vi "Phasor Compute Gated Phasor.vi"(7 "Phasor Calculation Type":T1, 8 "Error In":errorcluster, 9 "j 2 pi f":cxt, 10 "Gates Definitions":T4={"First Gate: t1"=0.0, "Gate Width: W"=0.0, "Gate Step: d"=0.0, "# Gates: G"=0.0, "Use Gate Center"=FALSE, "Frames/Image: F"=50, "Gates/Frame: L"=0, "Bits/Frame: q"=0, "Multiplicity: p"=0, "Gate Type"=enum."Square", "Gate Edge s"=4.0, "Gate Top Slope"=4.0, "Reversed Sawtooth?"=FALSE, "Computation"=FALSE, "User-defined Gate"={"X Array"=[], "Y Array"=[]}, "Tolerance"=50.0, "Integration"=enum."Item 0", "# Steps"=50.0, "Type of User-defined Function"=enum."Gate"}, 11 "Decay Definition":T2={"offset: t0"=0.0, "period: T"=0.0, "lifetime: tau"=0.0, "Incident Signal: I"=0.5, "Normalized Decays"=FALSE, "IRF Model"=enum."Dirac", "IRF Parameter 1"=0.0, "Poisson Signal"=FALSE}) -> (0 "Error Out":errorcluster, 3 "phasor":cxt, 4 "CPU (s)":dbl)   [LabVIEW 2021, in "Phasor.lvlib"]
uses:
  Phasor.lvlib
  Phasor Gate Definitions.ctl
  Phasor Gate Type.ctl
  Graphs/XY Graph/XY Graph Plot Data.ctl
  Phasor Decay Definiton.ctl
  Phasor IRF Model.ctl
  Phasor Calculation Type.ctl
  013d9567-a06e-4633-918d-fb7b214fbd4f.vi
  a72c2c01-1e7c-47d2-97e3-0247e5e3b51b.vi
  5bfd5da1-96d5-4f5c-8101-185aed7e9c89.vi
  a72c2c01-1e7c-47d2-97e3-0247e5e3b51b.vi/8a80743f-1319-44c8-96b0-3ef8fc688731.vi
  a72c2c01-1e7c-47d2-97e3-0247e5e3b51b.vi/931f4f8f-d8c6-4056-833f-5c8fe97b24b9.vi
  Math/ix/ix (EXT).vi
  Math/Math.lvlib
  Graphs/XY Graph/XY Graph Add-Ons.lvlib
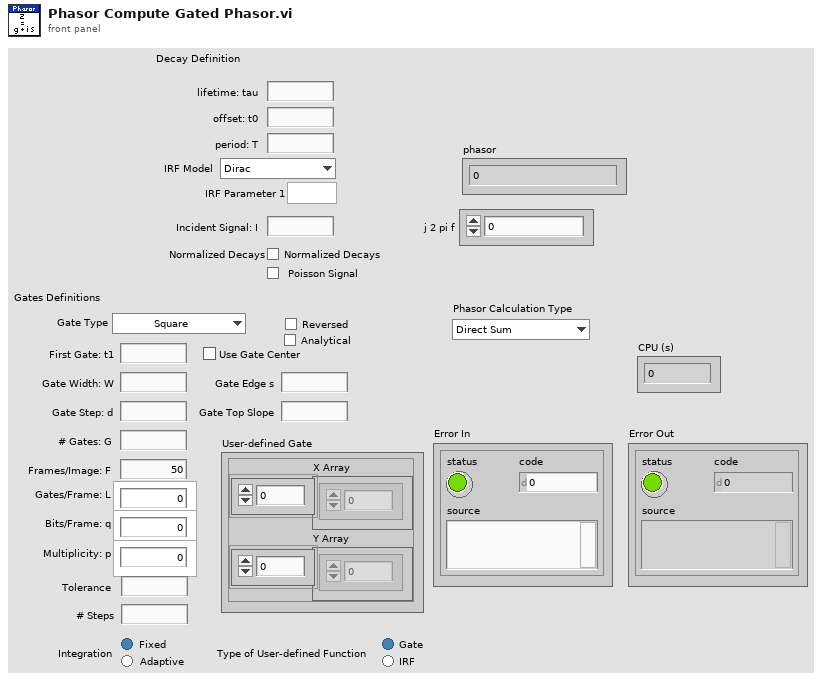
[diagram p1: front panel]
types:
  T1 = typedef "Phasor.lvlib/Phasor Calculation Type.ctl" = enum16{"Direct Sum", "Analytical Formula"}
  T2 = typedef "Phasor.lvlib/Phasor Decay Definiton.ctl" = cluster{"offset: t0":ext, "period: T":ext, "lifetime: tau":ext, "Incident Signal: I":ext, "Normalized Decays":bool, "IRF Model":T3, "IRF Parameter 1":ext, "Poisson Signal":bool}
  T3 = typedef "Phasor.lvlib/Phasor IRF Model.ctl" = enum16{"Dirac", "Exponential"}
  T4 = typedef "Phasor.lvlib/Phasor Gate Definitions.ctl" = cluster{"First Gate: t1":ext, "Gate Width: W":ext, "Gate Step: d":ext, "# Gates: G":ext, "Use Gate Center":bool, "Frames/Image: F":i32, "Gates/Frame: L":i32, "Bits/Frame: q":i32, "Multiplicity: p":i32, "Gate Type":T5, "Gate Edge s":ext, "Gate Top Slope":ext, "Reversed Sawtooth?":bool, "Computation":bool, "User-defined Gate":T6, "Tolerance":ext, "Integration":enum32{"Item 0", "Item 1"}, "# Steps":ext, "Type of User-defined Function":enum32{"Gate", "IRF"}}
  T5 = typedef "Phasor.lvlib/Phasor Gate Type.ctl" = enum16{"Square", "Finite Edge Square", "Finite Edge, Tilted Top Square", "Triangle", "Sawtooth", "User-defined"}
  T6 = typedef "XY Graph Add-Ons.lvlib/XY Graph Plot Data.ctl" = cluster{"X Array":dbl[], "Y Array":dbl[]}
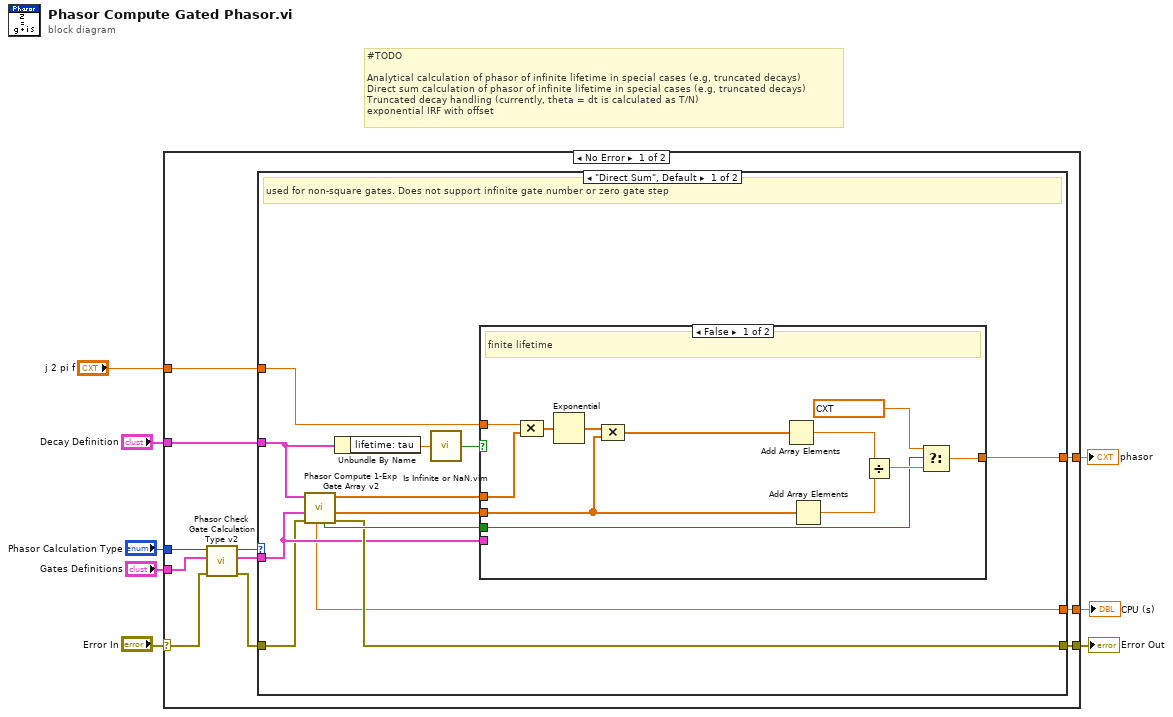
[diagram p0: block diagram]
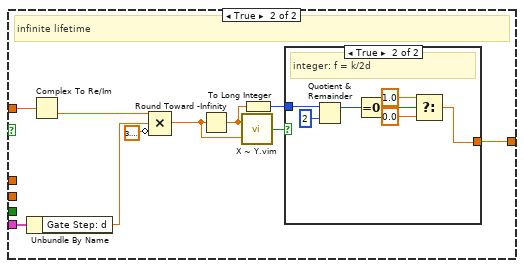
[diagram p2: hidden frame]
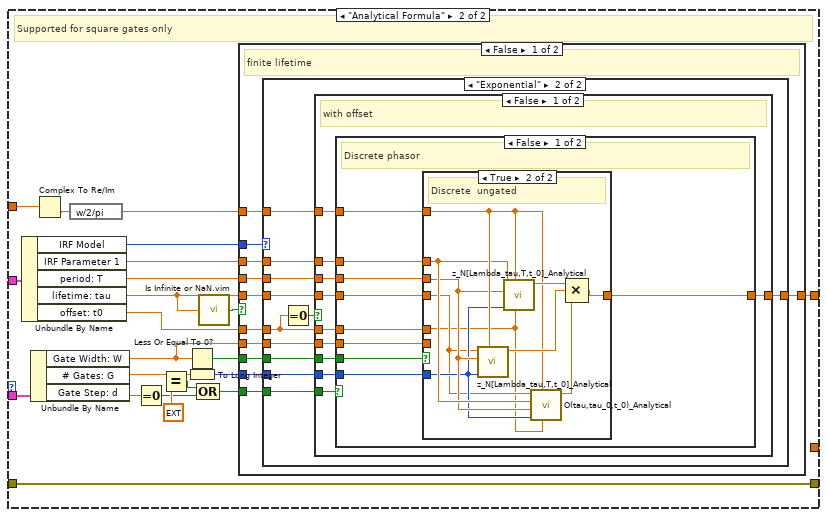
[diagram p4: hidden frame]
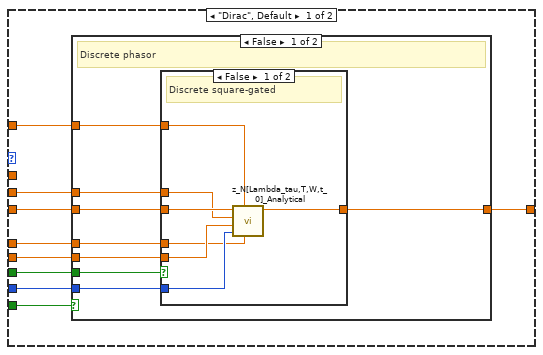
[diagram p5: hidden frame]
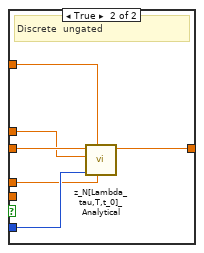
[diagram p6: hidden frame]
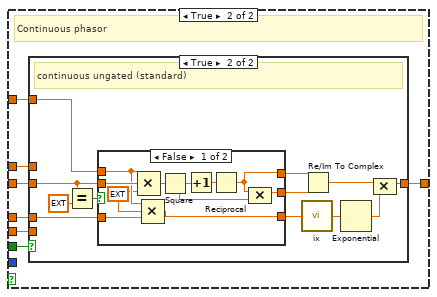
[diagram p7: hidden frame]
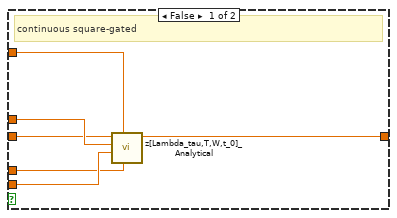
[diagram p8: hidden frame]
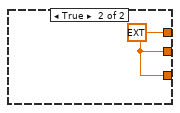
[diagram p9: hidden frame]
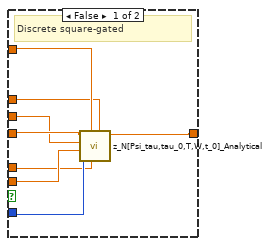
[diagram p10: hidden frame]
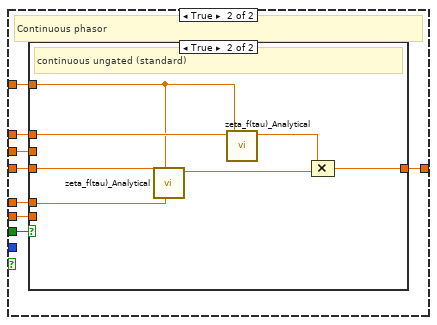
[diagram p11: hidden frame]
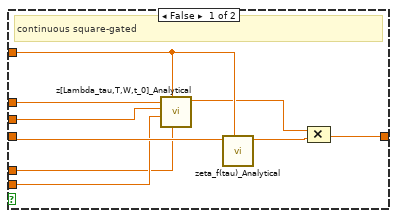
[diagram p12: hidden frame]
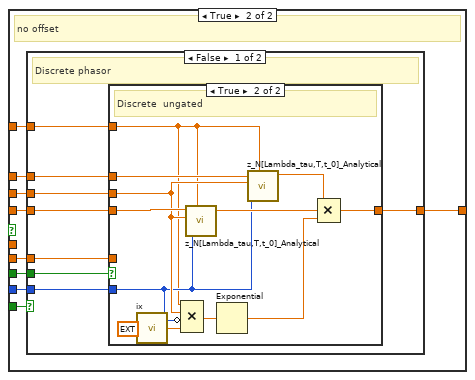
[diagram p13: hidden frame]
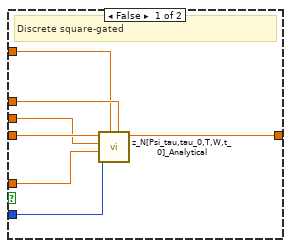
[diagram p14: hidden frame]
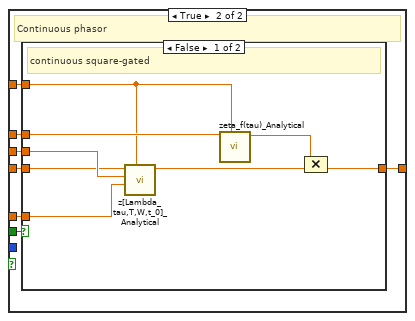
[diagram p15: hidden frame]
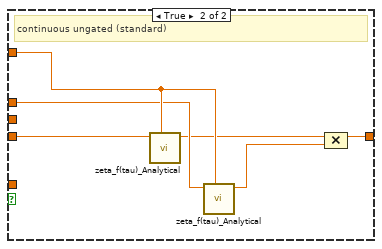
[diagram p16: hidden frame]
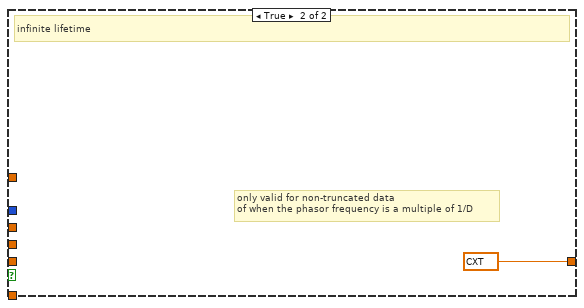
[diagram p17: hidden frame]
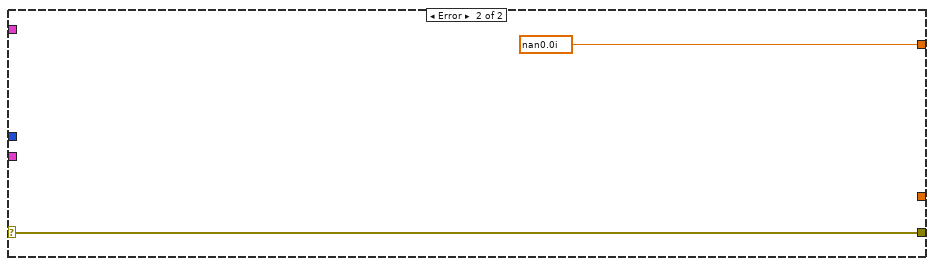
[diagram p18: hidden frame]
diagram:
  # "#TODO\n\nAnalytical calculation of phasor of infinite lifetime in special cases (e.g, truncated decays)\nDirect sum calculation of phasor of infinite lifetime in special cases (e.g, truncated decays)\nTruncated decay handling (currently, theta = dt is calculated as T/N)\nexponential IRF with offset"
  n1 = case shown="No Error" "Error In" {
    selector: "Error In" -> [w12 w291]
    tunnel: "Gates Definitions" -> [w13 _]
    tunnel: [w19 cdb nan+0.0i ("z")] -> w7
    tunnel: "Decay Definition" -> [w18 _]
    tunnel: "j 2 pi f" -> [w17 _]
    tunnel: "Phasor Calculation Type" -> [w14 _]
    tunnel: [w16 w291] -> w2
    tunnel: [w9 _] -> w1
    frame No Error {
      n2 = call "Phasor Check Gate Calculation Type v2.vi"("Error In"=w12, "Gates Definitions in"=w13, "Phasor Calculation Type in"=w14) -> ("Error Out"=w10:errorcluster, "Gates Definitions out"=w11:T4, "Phasor Calculation Type out"=w15:T1)  [unwired: 6 in]
      n3 = case shown="\"Direct Sum\", Default" w15 {
        tunnel: [w28 w78] -> w19
        tunnel: w18 -> [w24 w81]
        tunnel: w17 -> [w29 w80]
        tunnel: [w23 w61] -> w16
        tunnel: w11 -> [w22 w62]
        tunnel: w10 -> [w21 w61]
        tunnel: [w20 _] -> w9
        frame "Direct Sum", Default {
          # "used for non-square gates. Does not support infinite gate number or zero gate step"
          n4 = call "Phasor Compute 1-Exp Gate Array v2.vi"("Error In"=w21, "Gates Definitions"=w22, "Decay Definition"=w24) -> ("Error Out"=w23:errorcluster, "Gate Image Array"=w31:ext[], "t Array"=w30:ext[], "Small Gate Values?"=w27:bool, "CPU (s)"=w20:dbl)  [unwired: 4 in]
          n5 = Unbundle By Name(w24) -> ("lifetime: tau"=w26:ext)
          n6 = call "Is Infinite or NaN.vim"("Number"=w26) -> ("Is NaN or Inf?"=w25:bool)  [unwired: 8 in]
          n7 = case shown="False" w25 {
            tunnel: w31 -> [w41 _]
            tunnel: w30 -> [w38 _]
            tunnel: w29 -> [w37 w52]
            tunnel: [w35 w44] -> w28
            tunnel: w27 -> [w33 _]
            tunnel: w22 -> [_ w53]
            frame False {
              # "finite lifetime"
              n8 = Compound Arithmetic op=MULTIPLY(w37, w38) -> (w39:cxt[])
              n9 = Exponential(1:w39) -> (0:w40:cxt[])
              n10 = Compound Arithmetic op=MULTIPLY(w40, w41) -> (w36:cxt[])
              n11 = Add Array Elements(numeric array=w36) -> (sum=w42:cxt)
              n12 = Add Array Elements(numeric array=w41) -> (sum=w43:ext)
              n13 = Divide(x=w42, y=w43) -> (x/y=w34:cxt)
              n14 = Select(t=cxt nan+nani, s=w33, f=w34) -> (s? t:f=w35:cxt)
            }
            frame True {
              # "infinite lifetime"
              n15 = Unbundle By Name(w53) -> ("Gate Step: d"=w50:ext)
              n16 = Complex To Re/Im(x + iy=w52) -> (y=w51:ext)  [unwired: 1 out]
              n17 = Compound Arithmetic op=MULTIPLY(w51, w50, invert 3.141592653589793) -> (w48:ext)
              n18 = Round Toward -Infinity(1:w48) -> (0:w46:ext)
              n19 = call "X ~ Y.vim"("X"=w46, "Y"=w48) -> ("X ~= Y?"=w47:bool)  [unwired: 13 in]
              n20 = To Long Integer(number=w46) -> (32bit integer=w45:i32)
              n21 = case shown="True" w47 {
                tunnel: w45 -> [_ w60]
                tunnel: [_ w54] -> w44
                frame False {
                  # "not integer: f != k/2d"
                }
                frame True {
                  # "integer: f = k/2d"
                  n22 = Quotient & Remainder(x=w60, y=2) -> (x-y*floor(x/y)=w58:i32)  [unwired: 1 out]
                  n23 = Equal To 0?(x=w58) -> (x = 0?=w57:bool)
                  n24 = Select(t=1.0, s=w57, f=0.0) -> (s? t:f=w54:dbl)
                }
              }
            }
          }
        }
        frame "Analytical Formula" {
          # "Supported for square gates only"
          n25 = Unbundle By Name(w81) -> ("IRF Model"=w70:T3, "IRF Parameter 1"=w69:ext, "period: T"=w79:ext, "lifetime: tau"=w72:ext, "offset: t0"=w75:ext)
          n26 = Unbundle By Name(w62) -> ("Gate Width: W"=w77:ext, "# Gates: G"=w67:ext, "Gate Step: d"=w68:ext)
          n27 = Complex To Re/Im(x + iy=w80) -> (y=w73:ext)  [unwired: 1 out]
          n28 = expression code="w/2/pi"(w73) -> (w74:ext)
          n29 = Equal To 0?(x=w68) -> (x = 0?=w64:bool)
          n30 = Equal?(x=w67, y=ext inf) -> (x = y?=w65:bool)
          n31 = Less Or Equal To 0?(x=w77) -> (x <= 0?=w82:bool)
          n32 = To Long Integer(number=w67) -> (32bit integer=w76:i32)
          n33 = Compound Arithmetic op=OR(w65, w64) -> (w63:bool)
          n34 = call "Is Infinite or NaN.vim"("Number"=w72) -> ("Is NaN or Inf?"=w71:bool)  [unwired: 8 in]
          n35 = case shown="False" w71 {
            tunnel: w82 -> [w93 _]
            tunnel: w79 -> [w92 _]
            tunnel: [w91 cxt 0.0+0.0i ("z")] -> w78
            tunnel: w77 -> [w90 _]
            tunnel: w76 -> [w89 _]
            tunnel: w75 -> [w88 _]
            tunnel: w74 -> [w87 _]
            tunnel: w72 -> [w86 _]
            tunnel: w70 -> [w84 _]
            tunnel: w69 -> [w83 _]
            tunnel: w63 -> [w85 _]
            frame False {
              # "finite lifetime"
              n36 = case shown="\"Exponential\"" w84 {
                tunnel: w93 -> [w102 w170]
                tunnel: w92 -> [w101 w169]
                tunnel: [w100 w168] -> w91
                tunnel: w90 -> [w99 w167]
                tunnel: w89 -> [w98 w166]
                tunnel: w88 -> [w97 w161]
                tunnel: w87 -> [w96 w165]
                tunnel: w86 -> [w95 w164]
                tunnel: w85 -> [w94 w163]
                tunnel: w83 -> [_ w162]
                frame "Dirac", Default {
                  n37 = case shown="False" w94 {
                    tunnel: w102 -> [w110 w130]
                    tunnel: w96 -> [w107 w129]
                    tunnel: w101 -> [w108 w126]
                    tunnel: w95 -> [w109 w128]
                    tunnel: [w106 w127] -> w100
                    tunnel: w99 -> [w104 w125]
                    tunnel: w98 -> [w105 _]
                    tunnel: w97 -> [w103 w124]
                    frame False {
                      # "Discrete phasor"
                      n38 = case shown="False" w110 {
                        tunnel: w109 -> [w117 w123]
                        tunnel: w108 -> [w116 w122]
                        tunnel: w107 -> [w112 w119]
                        tunnel: [w113 w121] -> w106
                        tunnel: w105 -> [w114 w120]
                        tunnel: w104 -> [w115 _]
                        tunnel: w103 -> [w111 w118]
                        frame False {
                          # "Discrete square-gated"
                          n39 = call "z_N[Lambda_tau,T,W,t_0]_Analytical.vi"("t0"=w111, "Harmonic f"=w112, "N"=w114, "W"=w115, "T"=w116, "tau"=w117) -> ("z_n,N,W(tau)"=w113:cxt)  [unwired: 5 in]
                        }
                        frame True {
                          # "Discrete  ungated"
                          n40 = call "z_N[Lambda_tau,T,t_0]_Analytical.vi"("t0"=w118, "Harmonic f"=w119, "N"=w120, "T"=w122, "tau"=w123) -> ("z"=w121:cxt)  [unwired: 6 in]
                        }
                      }
                    }
                    frame True {
                      # "Continuous phasor"
                      n41 = case shown="True" w130 {
                        tunnel: w129 -> [w131 w148]
                        tunnel: w128 -> [w135 w141]
                        tunnel: [w133 w143] -> w127
                        tunnel: w126 -> [w136 _]
                        tunnel: w125 -> [w134 _]
                        tunnel: w124 -> [w132 w144]
                        frame False {
                          # "continuous square-gated"
                          n42 = call "z[Lambda_tau,T,W,t_0]_Analytical.vi"("t0"=w132, "Harmonic f"=w131, "W"=w134, "T"=w136, "tau"=w135) -> ("z"=w133:cxt)  [unwired: 6 in]
                        }
                        frame True {
                          # "continuous ungated (standard)"
                          n43 = Equal?(x=w141, y=ext inf) -> (x = y?=w138:bool)
                          n44 = case shown="False" w138 {
                            tunnel: [w151 w159] -> w147
                            tunnel: [w149 w159] -> w146
                            tunnel: w148 -> [w155 _]
                            tunnel: w141 -> [w158 _]
                            tunnel: w144 -> [w153 _]
                            tunnel: [w152 w159] -> w139
                            frame False {
                              w154 = ext 6.283185307179586477
                              n45 = Compound Arithmetic op=MULTIPLY(w155, w158, w154) -> (w150:ext)
                              n46 = Compound Arithmetic op=MULTIPLY(w155, w154, w153) -> (w152:ext)
                              n47 = Square(x=w150) -> (x^2=w157:ext)
                              n48 = Increment(x=w157) -> (x+1=w156:ext)
                              n49 = Reciprocal(x=w156) -> (1/x=w151:ext)
                              n50 = Compound Arithmetic op=MULTIPLY(w151, w150) -> (w149:ext)
                            }
                            frame True {
                              w159 = ext 0.0 ("Re")
                              # "tau = Inf"
                            }
                          }
                          n51 = call-poly "ix.vi"("x (1)"=w139) -> ("i.(x)"=w137:cxt)
                          n52 = Re/Im To Complex(1:w146, 2:w147) -> (0:w145:cxt)
                          n53 = Exponential(1:w137) -> (0:w142:cxt)
                          n54 = Compound Arithmetic op=MULTIPLY(w145, w142) -> (w143:cxt)
                        }
                      }
                    }
                  }
                }
                frame "Exponential" {
                  n55 = Equal To 0?(x=w161) -> (x = 0?=w160:bool)
                  n56 = case shown="False" w160 {
                    tunnel: w170 -> [w175 w240]
                    tunnel: w169 -> [w179 w239]
                    tunnel: [w173 w238] -> w168
                    tunnel: w167 -> [w176 w237]
                    tunnel: w166 -> [w172 w236]
                    tunnel: w165 -> [w180 w235]
                    tunnel: w164 -> [w178 w234]
                    tunnel: w163 -> [w174 w233]
                    tunnel: w162 -> [w171 w232]
                    tunnel: w161 -> [w177 _]
                    frame False {
                      # "with offset"
                      n57 = case shown="False" w174 {
                        tunnel: w175 -> [w189 w215]
                        tunnel: w180 -> [w186 w214]
                        tunnel: w179 -> [w187 w211]
                        tunnel: w178 -> [w188 w213]
                        tunnel: [w181 w212] -> w173
                        tunnel: w176 -> [w184 w210]
                        tunnel: w172 -> [w185 _]
                        tunnel: w177 -> [w183 w209]
                        tunnel: w171 -> [w182 w208]
                        frame False {
                          # "Discrete phasor"
                          n58 = case shown="True" w189 {
                            tunnel: w188 -> [w195 w199]
                            tunnel: w187 -> [w194 w201]
                            tunnel: w186 -> [w197 w203]
                            tunnel: w185 -> [w192 w200]
                            tunnel: w184 -> [w193 _]
                            tunnel: w183 -> [w191 w198]
                            tunnel: w182 -> [w196 w202]
                            tunnel: [w190 w205] -> w181
                            frame False {
                              # "Discrete square-gated"
                              n59 = call "z_N[Psi_tau,tau_0,T,W,t_0]_Analytical.vi"("tau_0"=w196, "t0"=w191, "Harmonic f"=w197, "N"=w192, "W"=w193, "T"=w194, "tau"=w195) -> ("z_n,N,W(tau,tau_0)"=w190:cxt)  [unwired: 4 in]
                            }
                            frame True {
                              # "Discrete  ungated"
                              n60 = call "z_N[Lambda_tau,T,t_0]_Analytical.vi"("Harmonic f"=w203, "N"=w200, "T"=w201, "tau"=w199) -> ("z"=w206:cxt)  [unwired: 7 in]
                              n61 = call "z_N[Lambda_tau,T,t_0]_Analytical.vi"("t0"=w198, "Harmonic f"=w203, "N"=w200, "T"=w201, "tau"=w202) -> ("z"=w207:cxt)  [unwired: 6 in]
                              n62 = call "O(tau,tau_0,t_0)_Analytical.vi"("t0"=w198, "Harmonic f"=w203, "N"=w200, "T"=w201, "tau_0"=w202, "tau"=w199) -> ("O(tau_tau_0,t_0)"=w204:cxt)  [unwired: 5 in]
                              n63 = Compound Arithmetic op=MULTIPLY(w207, w206, w204) -> (w205:cxt)
                            }
                          }
                        }
                        frame True {
                          # "Continuous phasor"
                          n64 = case shown="True" w215 {
                            tunnel: w214 -> [w222 w228]
                            tunnel: w213 -> [w224 w227]
                            tunnel: [w216 w230] -> w212
                            tunnel: w211 -> [w220 _]
                            tunnel: w210 -> [w219 _]
                            tunnel: w209 -> [w218 w225]
                            tunnel: w208 -> [w221 w229]
                            frame False {
                              # "continuous square-gated"
                              n65 = call "z[Lambda_tau,T,W,t_0]_Analytical.vi"("t0"=w218, "Harmonic f"=w222, "W"=w219, "T"=w220, "tau"=w221) -> ("z"=w217:cxt)  [unwired: 6 in]
                              n66 = call "zeta_f(tau)_Analytical.vi"("Harmonic f"=w222, "tau"=w224) -> ("z"=w223:cxt)  [unwired: 9 in]
                              n67 = Compound Arithmetic op=MULTIPLY(w217, w223) -> (w216:cxt)
                            }
                            frame True {
                              # "continuous ungated (standard)"
                              n68 = call "zeta_f(tau)_Analytical.vi"("t0"=w225, "Harmonic f"=w228, "tau"=w227) -> ("z"=w226:cxt)  [unwired: 8 in]
                              n69 = call "zeta_f(tau)_Analytical.vi"("Harmonic f"=w228, "tau"=w229) -> ("z"=w231:cxt)  [unwired: 9 in]
                              n70 = Compound Arithmetic op=MULTIPLY(w231, w226) -> (w230:cxt)
                            }
                          }
                        }
                      }
                    }
                    frame True {
                      # "no offset"
                      n71 = case shown="False" w233 {
                        tunnel: w240 -> [w248 w274]
                        tunnel: w235 -> [w245 w273]
                        tunnel: w239 -> [w246 w270]
                        tunnel: w234 -> [w247 w272]
                        tunnel: [w244 w271] -> w238
                        tunnel: w237 -> [w242 w269]
                        tunnel: w236 -> [w243 _]
                        tunnel: w232 -> [w241 w268]
                        frame False {
                          # "Discrete phasor"
                          n72 = case shown="True" w248 {
                            tunnel: w247 -> [w255 w267]
                            tunnel: w246 -> [w252 w261]
                            tunnel: w245 -> [w253 w256]
                            tunnel: [w249 w264] -> w244
                            tunnel: w243 -> [w250 w260]
                            tunnel: w242 -> [w251 _]
                            tunnel: w241 -> [w254 w265]
                            frame False {
                              # "Discrete square-gated"
                              n73 = call "z_N[Psi_tau,tau_0,T,W,t_0]_Analytical.vi"("tau_0"=w254, "Harmonic f"=w253, "N"=w250, "W"=w251, "T"=w252, "tau"=w255) -> ("z_n,N,W(tau,tau_0)"=w249:cxt)  [unwired: 5 in]
                            }
                            frame True {
                              # "Discrete  ungated"
                              n74 = call-poly "ix.vi"("x (1)"=ext 6.283185307179586477) -> ("i.(x)"=w257:cxt)
                              n75 = Compound Arithmetic op=MULTIPLY(w256, w261, invert w260, w257) -> (w259:cxt)
                              n76 = call "z_N[Lambda_tau,T,t_0]_Analytical.vi"("Harmonic f"=w256, "N"=w260, "T"=w261, "tau"=w267) -> ("z"=w266:cxt)  [unwired: 7 in]
                              n77 = Exponential(1:w259) -> (0:w258:cxt)
                              n78 = call "z_N[Lambda_tau,T,t_0]_Analytical.vi"("Harmonic f"=w256, "N"=w260, "T"=w261, "tau"=w265) -> ("z"=w263:cxt)  [unwired: 7 in]
                              n79 = Compound Arithmetic op=MULTIPLY(w263, w266, w258) -> (w264:cxt)
                            }
                          }
                        }
                        frame True {
                          # "Continuous phasor"
                          n80 = case shown="False" w274 {
                            tunnel: w273 -> [w277 w288]
                            tunnel: w272 -> [w281 w286]
                            tunnel: [w276 w287] -> w271
                            tunnel: w270 -> [w282 _]
                            tunnel: w269 -> [w280 _]
                            tunnel: w268 -> [w278 w285]
                            frame False {
                              # "continuous square-gated"
                              n81 = call "z[Lambda_tau,T,W,t_0]_Analytical.vi"("Harmonic f"=w277, "W"=w280, "T"=w282, "tau"=w281) -> ("z"=w279:cxt)  [unwired: 7 in]
                              n82 = call "zeta_f(tau)_Analytical.vi"("Harmonic f"=w277, "tau"=w278) -> ("z"=w275:cxt)  [unwired: 9 in]
                              n83 = Compound Arithmetic op=MULTIPLY(w275, w279) -> (w276:cxt)
                            }
                            frame True {
                              # "continuous ungated (standard)"
                              n84 = call "zeta_f(tau)_Analytical.vi"("Harmonic f"=w288, "tau"=w286) -> ("z"=w284:cxt)  [unwired: 9 in]
                              n85 = call "zeta_f(tau)_Analytical.vi"("Harmonic f"=w288, "tau"=w285) -> ("z"=w283:cxt)  [unwired: 9 in]
                              n86 = Compound Arithmetic op=MULTIPLY(w284, w283) -> (w287:cxt)
                            }
                          }
                        }
                      }
                    }
                  }
                }
              }
            }
            frame True {
              # "only valid for non-truncated data\nof when the phasor frequency is a multiple of 1/D"
              # "infinite lifetime"
            }
          }
        }
      }
    }
    frame Error {
    }
  }
  "phasor" <- w7
  "Error Out" <- w2
  "CPU (s)" <- w1
